vi "vector_stat.vi"(0 "Array":dbl[](array[numeric])) -> (1 "Average":dbl, 2 "Sigma":dbl)   [LabVIEW 2015]
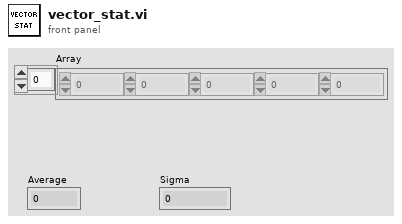
[diagram p1: front panel]
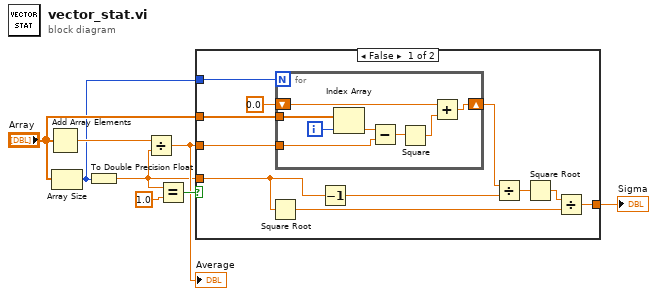
[diagram p0: block diagram]
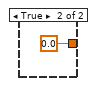
[diagram p2: hidden frame]
diagram:
  n1 = Add Array Elements(numeric array="Array") -> (sum=w8:dbl)
  n2 = Array Size(array="Array") -> (size(s)=w1:i32)
  n3 = To Double Precision Float(number=w1) -> (double precision float=w2:dbl)
  n4 = Divide(x=w8, y=w2) -> (x/y=w3:dbl)
  "Average" <- w3
  n5 = Equal?(x=w2, y=1.0) -> (x = y?=w6:bool)
  n6 = case shown="False" w6 {
    tunnel: [w11 0.0] -> w5
    tunnel: w2 -> [w9 _]
    tunnel: "Array" -> [w19 _]
    tunnel: w3 -> [w18 _]
    tunnel: w1 -> [w10 _]
    frame False {
      n7 = Square Root(x=w9) -> (sqrt(x)=w12:dbl)
      n8 = for {
        N: w10 -> [_]
        tunnel: w19 -> [w26]
        tunnel: w18 -> [w25]
        shift-right: [w20] -> w16
        shift-left: 0.0 -> [w22]
        i -> [w27]
        n9 = Index Array(array=w26, index=w27) -> (element=w24:dbl)
        n10 = Subtract(x=w24, y=w25) -> (x-y=w23:dbl)
        n11 = Square(x=w23) -> (x^2=w21:dbl)
        n12 = Add(x=w22, y=w21) -> (x+y=w20:dbl)
      }
      n13 = Decrement(x=w9) -> (x-1=w15:dbl)
      n14 = Divide(x=w16, y=w15) -> (x/y=w14:dbl)
      n15 = Square Root(x=w14) -> (sqrt(x)=w13:dbl)
      n16 = Divide(x=w13, y=w12) -> (x/y=w11:dbl)
    }
    frame True {
    }
  }
  "Sigma" <- w5
